vi "DaNI moving.vi"(9 "location":dbl[](array[numeric]), 10 "direction":string, 11 "Priority level array":dbl[][](array[numeric])) -> (2 "new direction":string, 3 "new location":dbl[](array[numeric]))   [LabVIEW 2015]
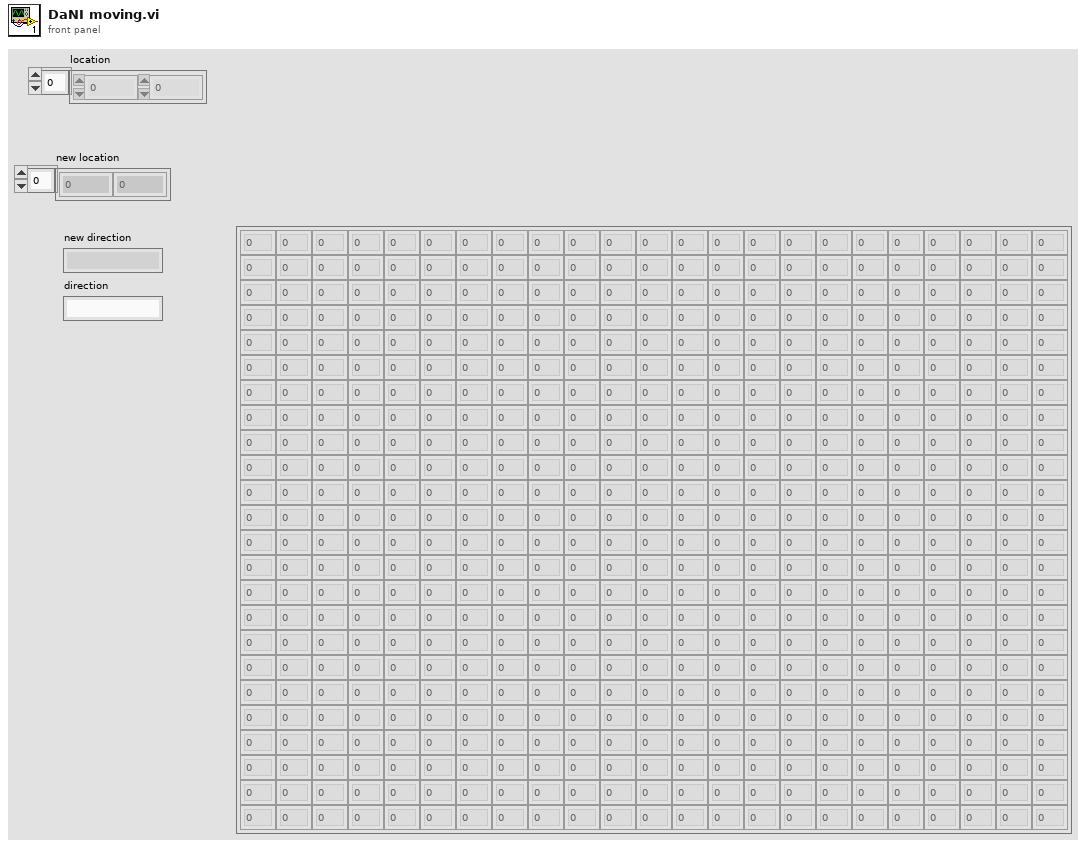
[diagram p1: front panel]
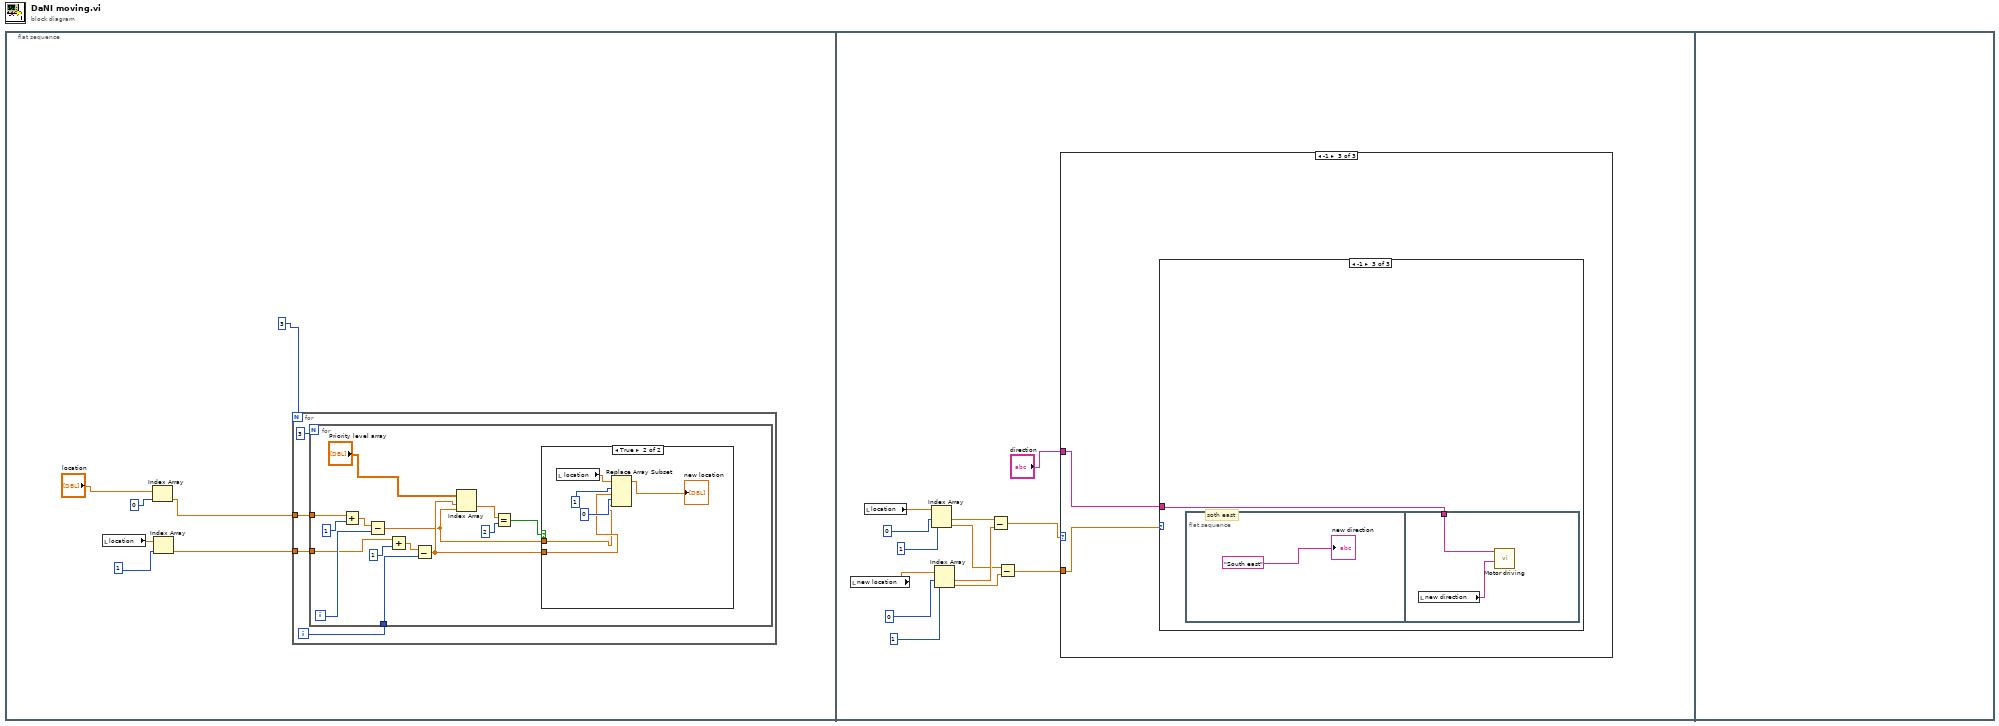
[diagram p0: block diagram]
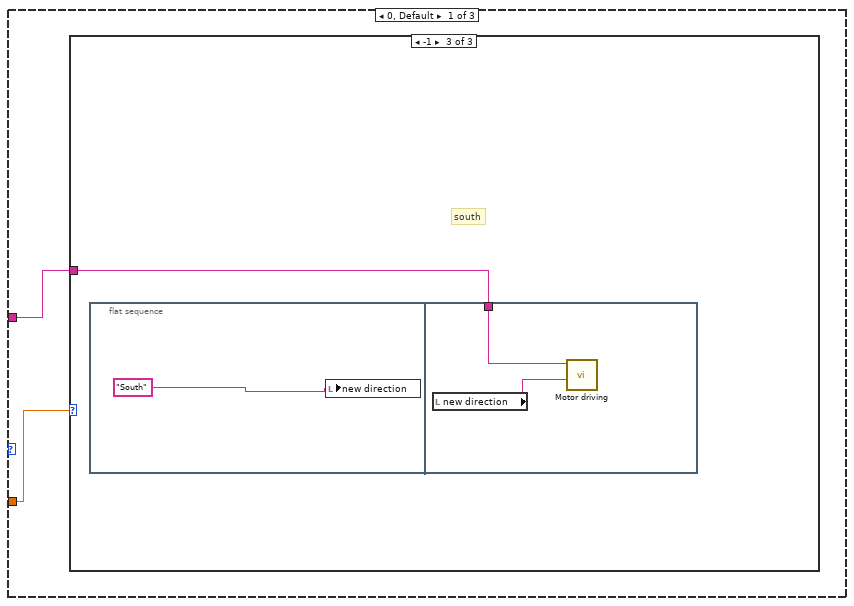
[diagram p3: hidden frame]
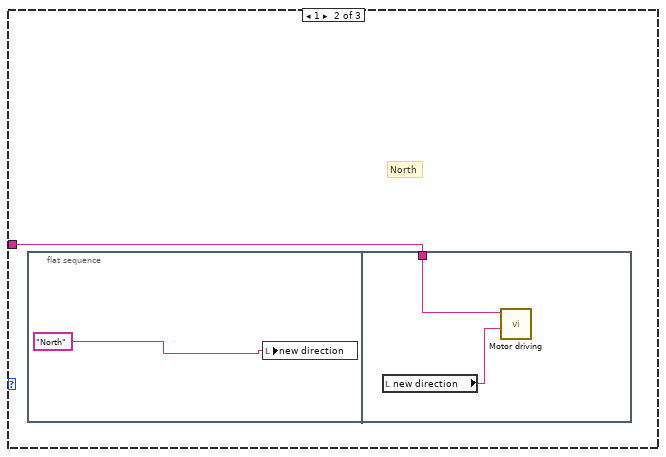
[diagram p5: hidden frame]
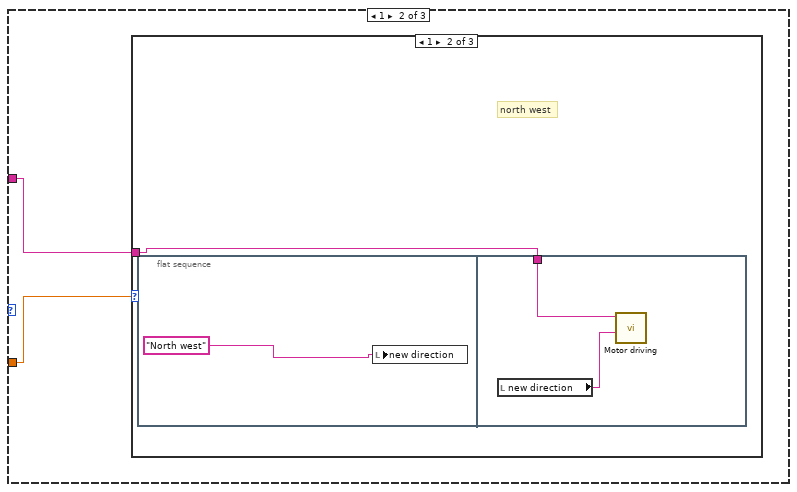
[diagram p6: hidden frame]
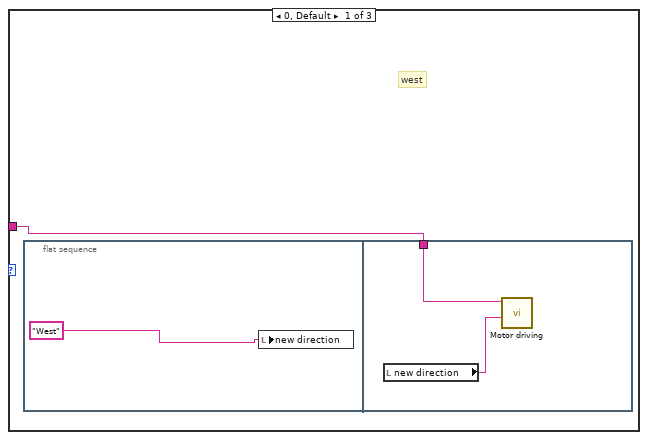
[diagram p7: hidden frame]
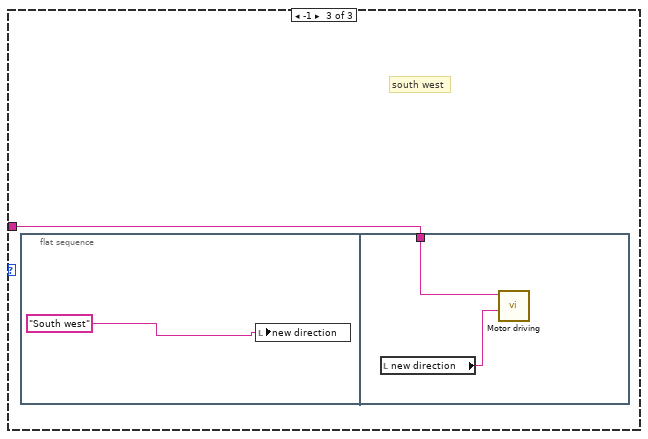
[diagram p8: hidden frame]
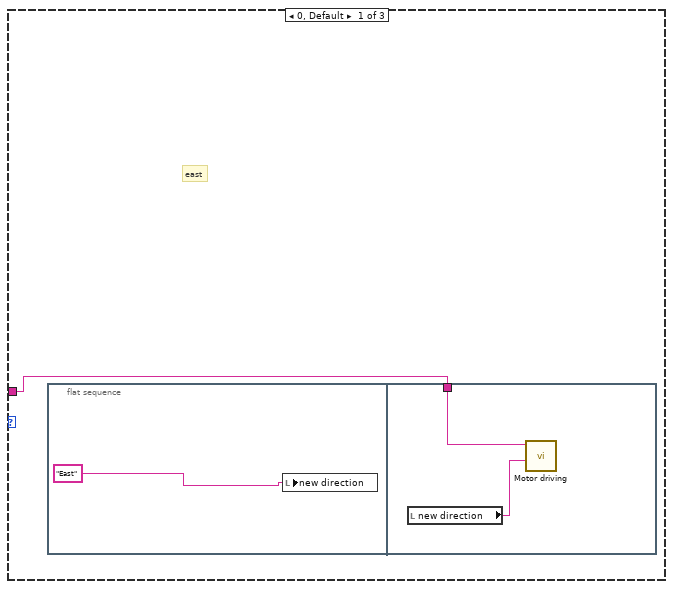
[diagram p9: hidden frame]
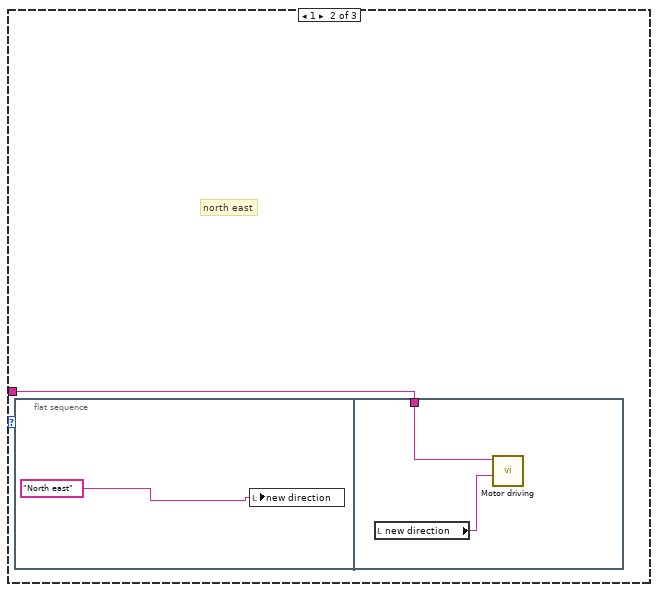
[diagram p10: hidden frame]
diagram:
  n1 = flat-sequence {
    frame #0 {
      n2 = local read "location"() -> (w6:dbl[])
      n3 = Index Array(array="location", index=0) -> (element=w3:dbl)
      n4 = Index Array(array=w6, index=1) -> (element=w2:dbl)
      n5 = for {
        N: 3 -> [_]
        tunnel: w3 -> [w9]
        tunnel: w2 -> [w8]
        i -> [w10]
        n6 = for {
          N: 3 -> [_]
          tunnel: w10 -> [w20]
          tunnel: w9 -> [w19]
          tunnel: w8 -> [w18]
          i -> [w23]
          n7 = Add(x=w19, y=1) -> (x+y=w24:dbl)
          n8 = Subtract(x=w24, y=w23) -> (x-y=w12:dbl)
          n9 = Add(x=w18, y=1) -> (x+y=w21:dbl)
          n10 = Subtract(x=w21, y=w20) -> (x-y=w14:dbl)
          n11 = Index Array(array="Priority level array", index (row)=w14, index (col)=w12) -> (element=w17:dbl)
          n12 = Equal?(x=w17, y=2) -> (x = y?=w15:bool)
          n13 = case shown="True" w15 {
            tunnel: w12 -> [_ w28]
            tunnel: w14 -> [_ w29]
            frame False {
            }
            frame True {
              n14 = local read "location"() -> (w27:dbl[])
              n15 = Replace Array Subset(array=w27, new element #1=w29, index #1=1, new element #2=w28, index #2=0) -> (→"new location":dbl[])
            }
          }
        }
      }
    }
    frame #1 {
      n16 = local read "new location"() -> (w41:dbl[])
      n17 = local read "location"() -> (w44:dbl[])
      n18 = Index Array(array=w44, index #1=0, index #2=1) -> (element #1=w38:dbl, element #2=w36:dbl)
      n19 = Index Array(array=w41, index #1=0, index #2=1) -> (element #1=w37:dbl, element #2=w35:dbl)
      n20 = Subtract(x=w38, y=w37) -> (x-y=w33:dbl)
      n21 = Subtract(x=w36, y=w35) -> (x-y=w34:dbl)
      n22 = case shown="-1" w33 {
        tunnel: w34 -> [w46 w56 w70]
        tunnel: "direction" -> [w45 w55 w69]
        frame 0, Default {
          n23 = case shown="-1" w46 {
            tunnel: w45 -> [_ w47 w51]
            frame 0, Default {
              # "Nothing"
            }
            frame 1 {
              # "North"
              n24 = flat-sequence {
                tunnel: w47 -> [w50]
                frame #0 {
                  n25 = local write "new direction"("North") -> ()
                }
                frame #1 {
                  n26 = local read "new direction"() -> (w49:string)
                  n27 = call "Motor driving.vi"("New direction"=w49, "Current direction"=w50) -> ()  [unwired: 10 in]
                }
              }
            }
            frame -1 {
              # "south"
              n28 = flat-sequence {
                tunnel: w51 -> [w53]
                frame #0 {
                  n29 = local write "new direction"("South") -> ()
                }
                frame #1 {
                  n30 = local read "new direction"() -> (w54:string)
                  n31 = call "Motor driving.vi"("New direction"=w54, "Current direction"=w53) -> ()  [unwired: 10 in]
                }
              }
            }
          }
        }
        frame 1 {
          n32 = case shown="1" w56 {
            tunnel: w55 -> [w57 w61 w65]
            frame 0, Default {
              # "west"
              n33 = flat-sequence {
                tunnel: w57 -> [w60]
                frame #0 {
                  n34 = local write "new direction"("West") -> ()
                }
                frame #1 {
                  n35 = local read "new direction"() -> (w59:string)
                  n36 = call "Motor driving.vi"("New direction"=w59, "Current direction"=w60) -> ()  [unwired: 10 in]
                }
              }
            }
            frame 1 {
              # "north west"
              n37 = flat-sequence {
                tunnel: w61 -> [w64]
                frame #0 {
                  n38 = local write "new direction"("North west") -> ()
                }
                frame #1 {
                  n39 = local read "new direction"() -> (w63:string)
                  n40 = call "Motor driving.vi"("New direction"=w63, "Current direction"=w64) -> ()  [unwired: 10 in]
                }
              }
            }
            frame -1 {
              # "south west"
              n41 = flat-sequence {
                tunnel: w65 -> [w68]
                frame #0 {
                  n42 = local write "new direction"("South west") -> ()
                }
                frame #1 {
                  n43 = local read "new direction"() -> (w67:string)
                  n44 = call "Motor driving.vi"("New direction"=w67, "Current direction"=w68) -> ()  [unwired: 10 in]
                }
              }
            }
          }
        }
        frame -1 {
          n45 = case shown="-1" w70 {
            tunnel: w69 -> [w71 w75 w79]
            frame 0, Default {
              # "east"
              n46 = flat-sequence {
                tunnel: w71 -> [w74]
                frame #0 {
                  n47 = local write "new direction"("East") -> ()
                }
                frame #1 {
                  n48 = local read "new direction"() -> (w73:string)
                  n49 = call "Motor driving.vi"("New direction"=w73, "Current direction"=w74) -> ()  [unwired: 10 in]
                }
              }
            }
            frame 1 {
              # "north east"
              n50 = flat-sequence {
                tunnel: w75 -> [w78]
                frame #0 {
                  n51 = local write "new direction"("North east") -> ()
                }
                frame #1 {
                  n52 = local read "new direction"() -> (w77:string)
                  n53 = call "Motor driving.vi"("New direction"=w77, "Current direction"=w78) -> ()  [unwired: 10 in]
                }
              }
            }
            frame -1 {
              # "soth east"
              n54 = flat-sequence {
                tunnel: w79 -> [w82]
                frame #0 {
                  "new direction" <- "South east"
                }
                frame #1 {
                  n55 = local read "new direction"() -> (w81:string)
                  n56 = call "Motor driving.vi"("New direction"=w81, "Current direction"=w82) -> ()  [unwired: 10 in]
                }
              }
            }
          }
        }
      }
    }
    frame #2 {
    }
  }
